vi "Parse Device IDs.vi"(8 "Error In":errorcluster, 9 "Data":string, 10 "Structure ID":string, 11 "Nest Config":T1) -> (0 "Error Out":errorcluster, 1 "Data":string, 2 "Device IDs":string[](array[string]), 3 "Nest Config":T1)   [LabVIEW 2013, in "LMH-Nest.lvlib"]
doc: "Parse device IDs from structure."
uses:
  LMH-Nest.lvlib
  Type Defs/Nest Config.ctl
  <vilib>/httpClient/ClientHandle.ctl
  Type Defs/Session Data.ctl
  <vilib>/httpClient/LabVIEWHTTPClient.lvlib
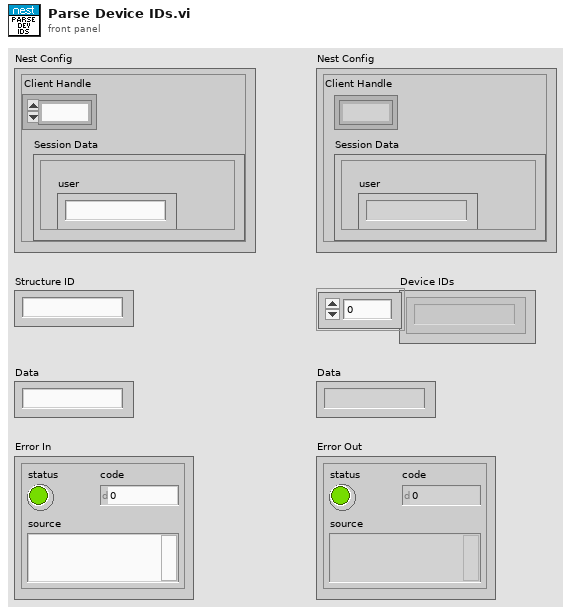
[diagram p1: front panel]
types:
  T1 = typedef "LMH-Nest.lvlib/Nest Config.ctl" = cluster{"Client Handle":T2, "Session Data":T3}
  T2 = typedef "LabVIEWHTTPClient.lvlib/ClientHandle.ctl" = refnum<k1>
  T3 = typedef "LMH-Nest.lvlib/Session Data.ctl" = cluster{"is_superuser":bool, "is_staff":bool, "urls":cluster{"transport_url":string, "rubyapi_url":string, "weather_url":string, "log_upload_url":string, "support_url":string}, "limits":cluster{"thermostats_per_structure":u32, "structures":u32, "thermostats":u32, "smoke_detectors":u32, "smoke_detectors_per_structure":u32}, "access_token":string, "userid":string, "expires_in":string, "email":string, "user":string, "language":string}
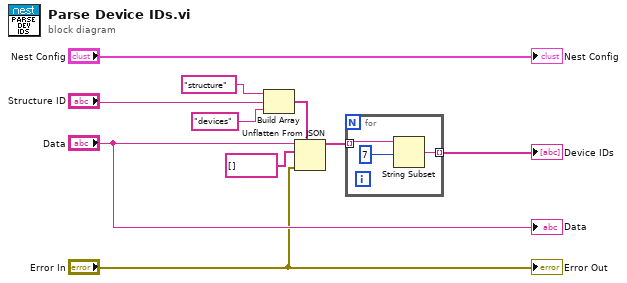
[diagram p0: block diagram]
diagram:
  n1 = Build Array("structure", "Structure ID", "devices" ("element")) -> (w6:string[])
  n2 = Unflatten From JSON(path=w6, JSON string="Data", type and defaults=string[] [], error in (no error)="Error In") -> (value=w3:string[])  [unwired: 3 in, 1 out]
  n3 = for {
    tunnel: w3 -> [w13] mode=indexing
    tunnel: [w11] -> w2 mode=indexing
    n4 = String Subset(string=w13, offset (0)=7) -> (substring=w11:string)  [unwired: 1 in]
  }
  "Device IDs" <- w2
  "Nest Config" <- "Nest Config"
  "Error Out" <- "Error In"
  "Data" <- "Data"
